vi "Feature Subset Selection (GA).vi"() -> ()   [LabVIEW 2016]
uses:
  _vlib/GA_tParameters.ctl
  4. Accuracy Assessment for EEG Classification/_vlib/CU_ClassifierTypes.ctl
  <vilib>/Math Plots/2D Math Plots/2D Error Bar/2D Error Bar XCtrl/2D Error Bar.xctl
  4. Accuracy Assessment for EEG Classification/_vlib/CU_ClassifierQualityMeasure.ctl
  _vlib/GA_metaParameters.ctl
  <vilib>/vision/Classification.llb/IMAQ SVM Kernel Options.ctl
  <vilib>/Math Plots/2D Math Plots/2D Error Bar/2D Error Bar Datatype/Public/Plot Helper (Fixed).vi
  4. Accuracy Assessment for EEG Classification/Classifier.lvlib
  _vlib/GA.lvlib
  <vilib>/Math Plots/2D Math Plots/2D Error Bar/2D Error Bar Datatype/2D Error Bar Datatype.lvclass
  <vilib>/Analysis/NI_AALBase.lvlib
panel:
  in  "Stop Button":bool
  in  "Tab Control":T1(tab)
  in  "ClassifierQualityMeasure":T2 caption="Критерий оценки точности классификации"
  in  "Use equal number of trials?":bool caption="Включить балансировку классов?"
  in  "Classifier Metaparameter":dbl=5.0 caption="Свободный параметр классификатора" min=0.0 max=100.0 step=0.1 format="%#_2g"
  in  "Iterations Num":i32=5
  in  "Training data paths":path[](array[path]) caption="Пути к файлам с обучающими данными"
  in  "Test data paths":path[](array[path]) caption="Пути к файлам с тестовыми данными"
  in  "True labels for Test data":path[](array[path]) caption="Пути к файлам с метками классов (для тестовых данных)"
  in  "Parameters":T3={"Population size"=100, "Generations no."=20, "Crossover probabality"=0.85, "Mutation mode"=enum."one-point, fixed rate", "Creep mutation"=FALSE, "Mutation rate"=0.05, "Min mutation rate"=0.0005, "Max mutation rate"=0.25, "Relative fitness differential"=1.0, "Reproduction plan"=enum."Steady-state-replace-worst", "Elitism"=FALSE, "FeaturesPerChannel"=5} caption="Параметры генетического алгоритма" {"Relative fitness differential" min=0.0 max=1.0; "Max mutation rate" min=0.0 max=1.0; "Min mutation rate" min=0.0 max=1.0; "Mutation rate" min=0.0 max=1.0; "Crossover probabality" min=0.0 max=1.0; "Generations no." min=1; "Population size" min=1}
  in  "ClassifierType":T4=enum."k NN Classifier" caption="Тип классификатора"
  in  "Start GA":bool
  out "Dataset Num":i32
  out "Total Progress":i32(slide) scale=0.0..25.0
  out "Solution":i32(listbox) caption="Решения, полученные после запусков ГА"
  out "Fitness Chart":cluster{i32[], dbl[]}[](graph) caption="Графики точности классификации"
  out "Accuracies":i32(listbox) caption="Оценки точности классификации на итерациях ГА"
  out "Iteration":i32
  out "Results":string caption="Протокол выполнения программы"
  out "Accuracies out":dbl[][](array[numeric]) caption="Результаты"
  out "2D Error Bar":refnum<class "2D Plot Datatype.lvclass">[](xcontrol) caption="График средней точности классификации"
  # "This VI is a part of BCI Design library, http://www.ru-bci.org \nCopyright © 2020, Sotnikov Peter, All rights reserved. License: GNU GPLv3"
  # "Число запусков ГА для каждого набора данных"
  # "Размер популяции"
  # "Число поколений"
  # "Вероятность скрещивания (кроссовера)"
  # "Тип мутации"
  # "Вероятность мутации"
  # "Значение nu для SVM-классификатора (0,0 .. 1,0)\nЧисло соседей k для kNN-классификатора (1 .. 100)\nЧисло нейронов N скрытого слоя для многослойного персептрона (1 .. 100)"
  # "Минимальная вероятность мутации"
  # "Максимальная вероятность мутации"
  # "Способ включения потомков в популяцию"
  # "Использовать элитизм?"
  # "Общее выполнение"
  # "Набор данных №"
  # "Запуск ГА №"
  # "Среднее \nпо наборам"
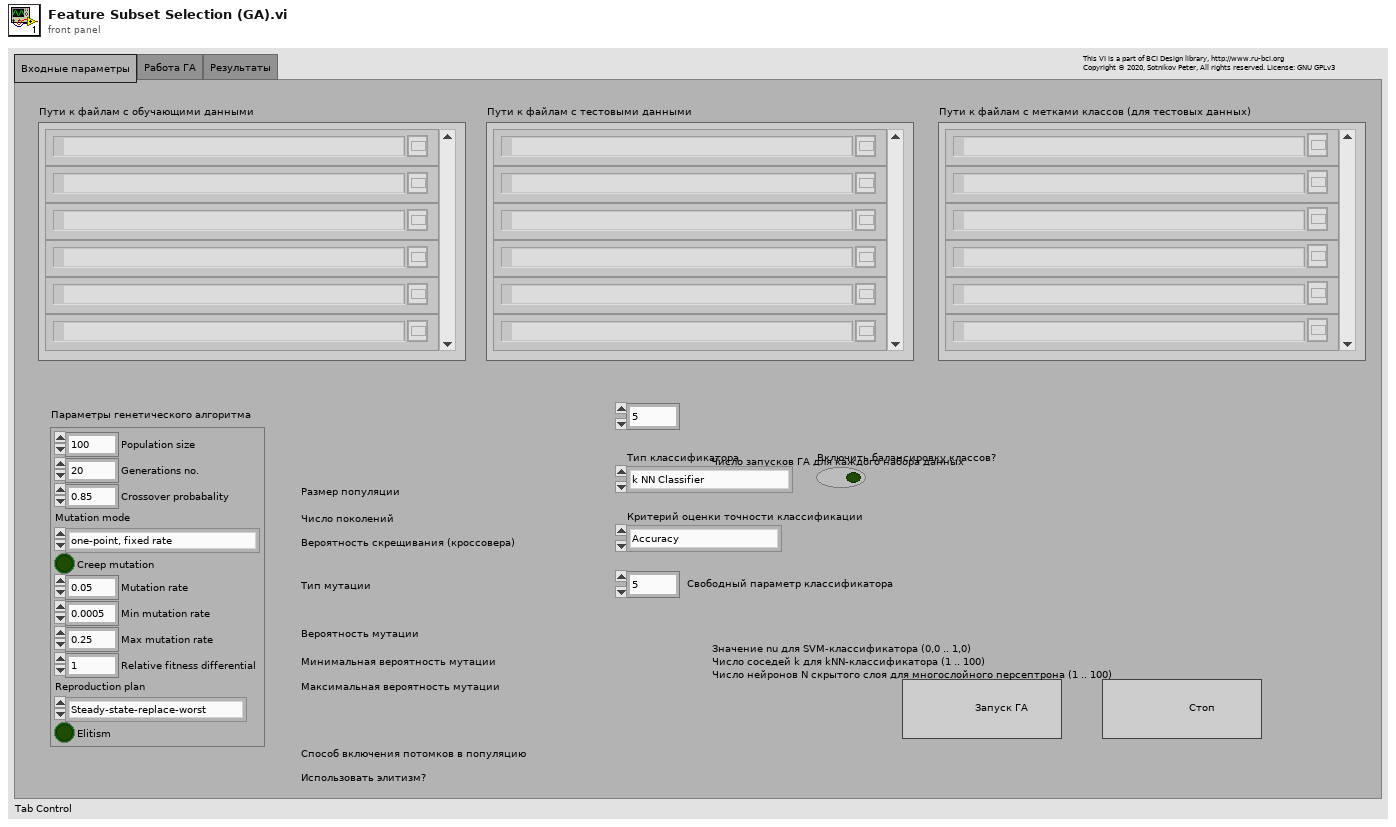
[diagram p1: front panel]
types:
  T1 = enum32{"Входные параметры", "Работа ГА", "Результаты"}
  T2 = typedef "Classifier.lvlib/CU_ClassifierQualityMeasure.ctl" = enum16{"Accuracy", "Cohen's kappa"}
  T3 = typedef "GA.lvlib/GA_tParameters.ctl" = cluster{"Population size":i32, "Generations no.":i32, "Crossover probabality":dbl, "Mutation mode":enum16{"one-point, fixed rate", "one-point, fitness-adjustable rate", "one-point, distance-adjustable rate"}, "Creep mutation":bool, "Mutation rate":dbl, "Min mutation rate":dbl, "Max mutation rate":dbl, "Relative fitness differential":dbl, "Reproduction plan":enum16{"Full generational replacement", "Steady-state-replace-random", "Steady-state-replace-worst"}, "Elitism":bool, "FeaturesPerChannel":i32}
  T4 = typedef "Classifier.lvlib/CU_ClassifierTypes.ctl" = enum16{"Multilayer perceptron", "k NN Classifier", "SVM Committee", "Mahalanobis distance", "SVM Classifier"}
  T5 = typedef "GA.lvlib/GA_metaParameters.ctl" = cluster{"Training Data Path":path, "Test Data Path":path, "True Labels for Test Trials":path, "ClassifierType":T4, "SVM Options":T6, "GA Parameters":T3, "Use equal number of trials?":bool, "Classifier Metaparameter":dbl, "ClassifierQualityMeasure":T2}
  T6 = typedef "IMAQ SVM Kernel Options.ctl" = cluster{"Kernel":enum32{"Linear", "Polynomial", "Gaussian", "RBF"}, "Degree":i32, "Gamma":dbl, "Coefficient":dbl, "Sigma":dbl, "Cache(MB)":dbl}
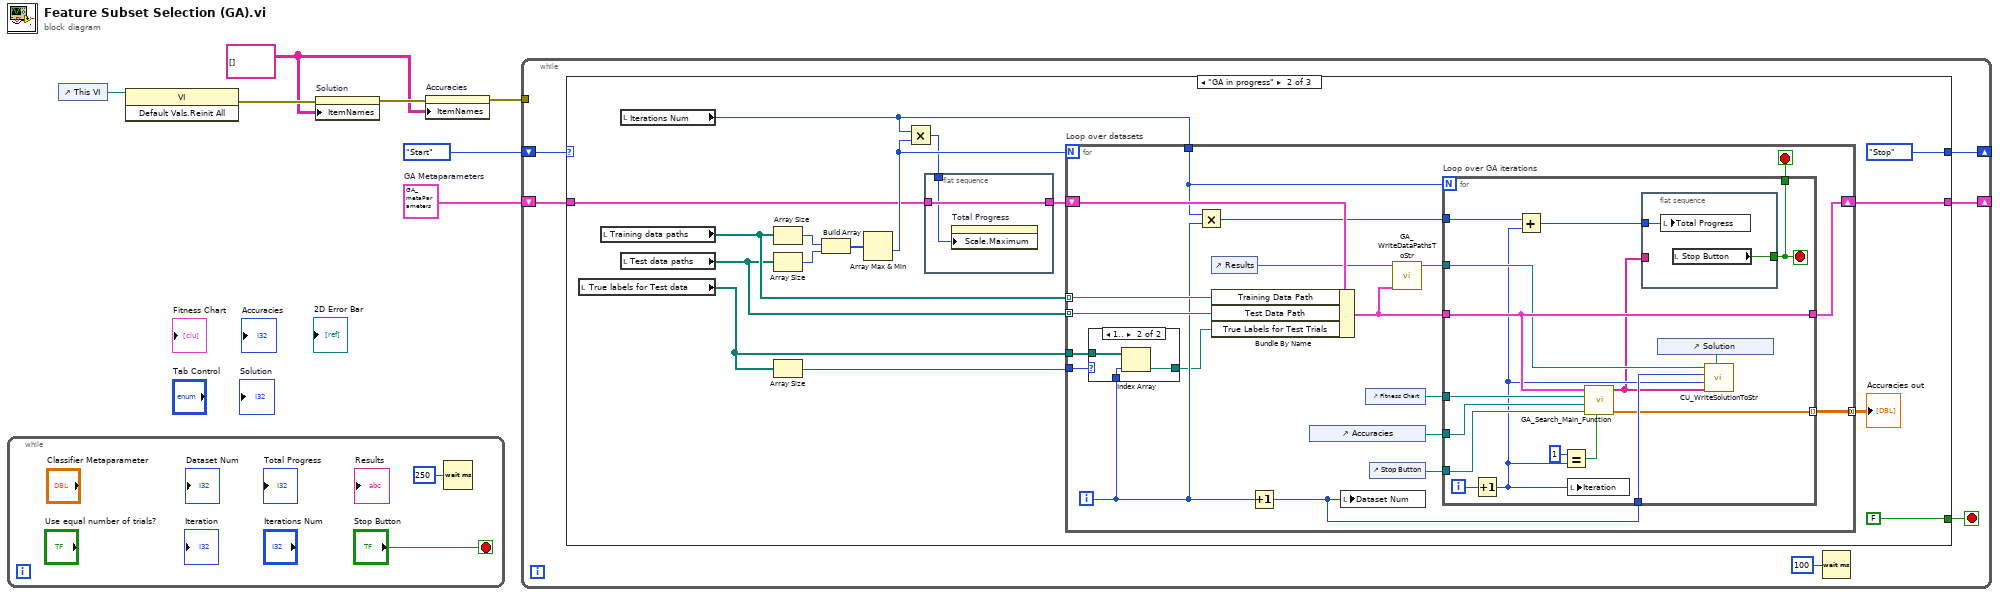
[diagram p0: block diagram]
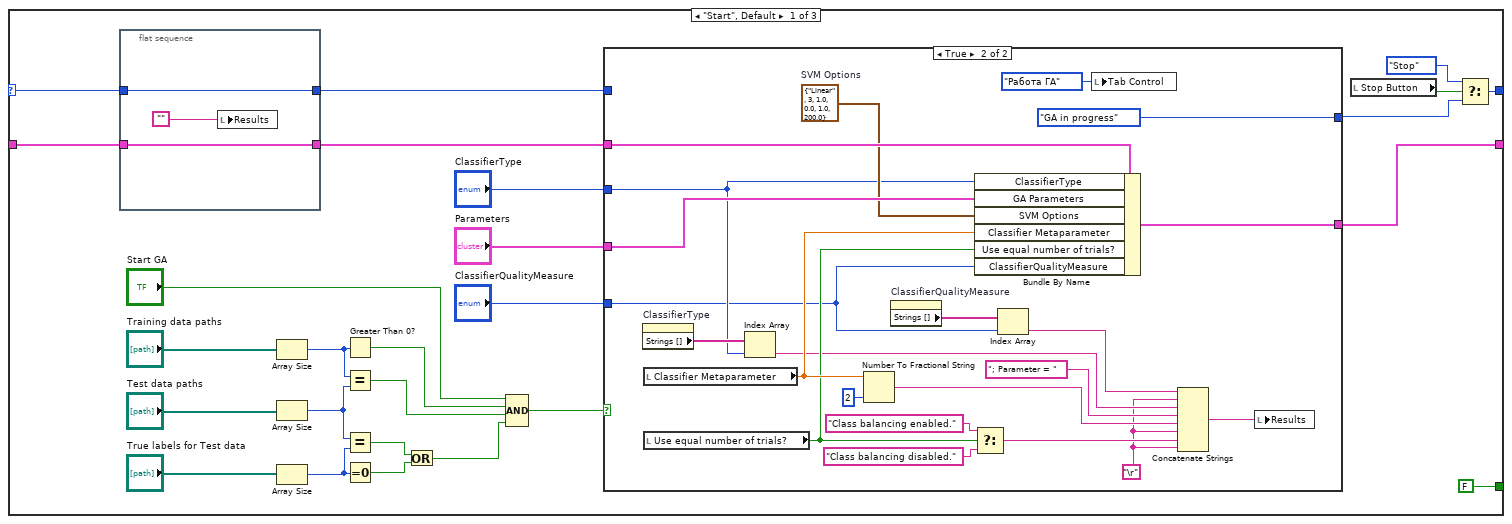
[diagram p2: hidden frame]
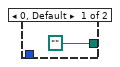
[diagram p4: hidden frame]
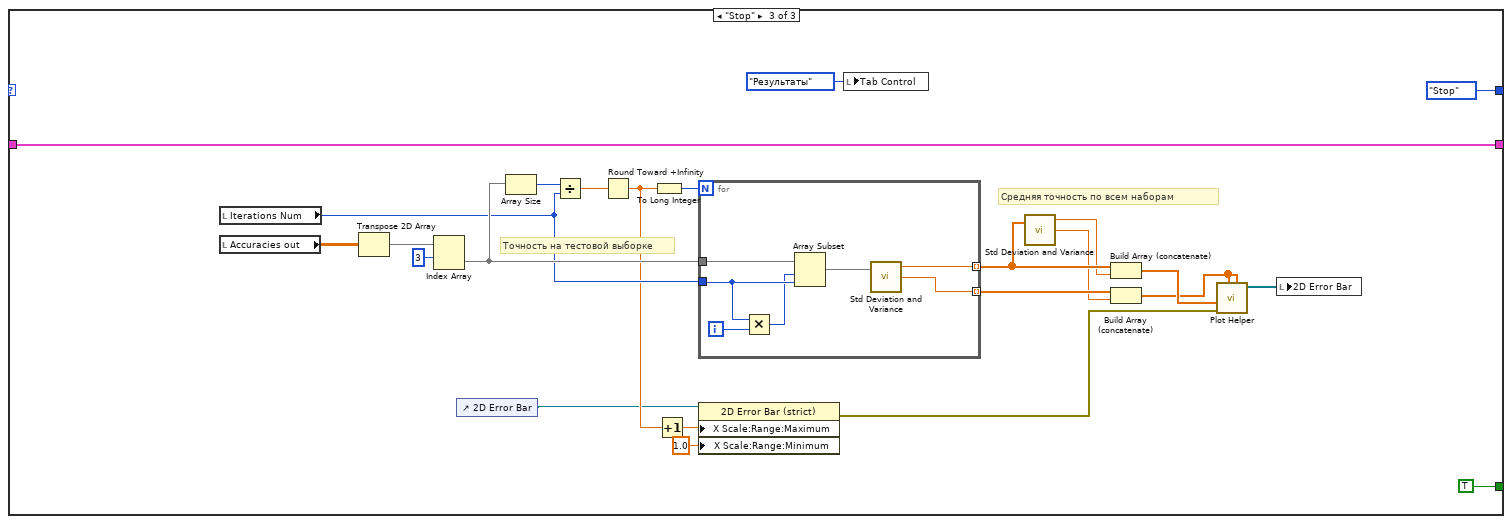
[diagram p5: hidden frame]
diagram:
  w1 = string[][] [] ("Item Names")
  w6 = T5 {"Training Data Path"=path "", "Test Data Path"=path "", "True Labels for Test Trials"=path "", "ClassifierType"=enum."Multilayer perceptron", "SVM Options"={"Kernel"=enum."Linear", "Degree"=0, "Gamma"=0.0, "Coefficient"=0.0, "Sigma"=0.0, "Cache(MB)"=0.0}, "GA Parameters"={"Population size"=0, "Generations no."=0, "Crossover probabality"=0.0, "Mutation mode"=enum."one-point, fixed rate", "Creep mutation"=FALSE, "Mutation rate"=0.0, "Min mutation rate"=0.0, "Max mutation rate"=0.0, "Relative fitness differential"=0.0, "Reproduction plan"=enum."Full generational replacement", "Elitism"=FALSE, "FeaturesPerChannel"=0}, "Use equal number of trials?"=FALSE, "Classifier Metaparameter"=5.0, "ClassifierQualityMeasure"=enum."Accuracy"}  # GA Metaparameters
  n1 = while {
    stop <- "Stop Button" stop-if-true
    n2 = Wait (ms)(milliseconds to wait=u32 250) -> ()  [unwired: 1 out]
  }
  n3 = control-ref of="This VI"() -> (w5:refnum<vi>)
  n4 = invoke class="VI" method="Default Vals.Reinit All"(reference=w5) -> (error out=w4:errorcluster)  [unwired: 2 in, 2 out]
  n5 = property on="Solution" class="MCListbox (strict)"(error in=w4, "ItemNames"=w1) -> (error out=w3:errorcluster)  [unwired: 1 in, 1 out]
  n6 = property on="Accuracies" class="MCListbox (strict)"(error in=w3, "ItemNames"=w1) -> (error out=w2:errorcluster)  [unwired: 1 in, 1 out]
  n7 = while {
    shift-right: [w12] -> _
    shift-left: w6 -> [w14]
    shift-right: [w13] -> _
    shift-left: enum16{"Start", "GA in progress", "Stop"}."Start" -> [w15]
    tunnel: w2 -> [_]
    stop <- w10 stop-if-true
    n8 = case shown="\"GA in progress\"" w15 {
      selector: w15 -> [w27 _ _]
      tunnel: w14 -> [w25 w70 w149]
      tunnel: [w31 enum16{"Start", "GA in progress", "Stop"}."Stop" ("t") enum16{"Start", "GA in progress", "Stop"}."Stop"] -> w13
      tunnel: [w33 w76 w149] -> w12
      tunnel: [FALSE FALSE TRUE] -> w10
      frame "Start", Default {
        n9 = flat-sequence {
          tunnel: w27 -> [w44]
          tunnel: [w44] -> w26
          tunnel: w25 -> [w43]
          tunnel: [w43] -> w24
          frame #0 {
            n10 = local write "Results"("") -> ()
          }
        }
        n11 = Array Size(array="Training data paths") -> (size(s)=w23:i32)
        n12 = Array Size(array="Test data paths") -> (size(s)=w41:i32)
        n13 = Array Size(array="True labels for Test data") -> (size(s)=w22:i32)
        n14 = Greater Than 0?(x=w23) -> (x > 0?=w17:bool)
        n15 = Equal?(x=w23, y=w41) -> (x = y?=w18:bool)
        n16 = Equal?(x=w41, y=w22) -> (x = y?=w21:bool)
        n17 = Equal To 0?(x=w22) -> (x = 0?=w20:bool)
        n18 = Or(x=w21, y=w20) -> (x .or. y?=w19:bool)
        n19 = Compound Arithmetic op=AND("Start GA", w17, w18, w19) -> (w40:bool)
        n20 = case shown="True" w40 {
          tunnel: w24 -> [w46 w68]
          tunnel: "ClassifierType" -> [_ w61]
          tunnel: "Parameters" -> [_ w67]
          tunnel: w26 -> [w45 _]
          tunnel: [w45 enum16{"Start", "GA in progress", "Stop"}."GA in progress"] -> w29
          tunnel: [w46 w64] -> w33
          tunnel: "ClassifierQualityMeasure" -> [_ w48]
          frame False {
          }
          frame True {
            w50 = "\r"
            w66 = T6 {"Kernel"=enum."Linear", "Degree"=3, "Gamma"=1.0, "Coefficient"=0.0, "Sigma"=1.0, "Cache(MB)"=200.0}  # SVM Options
            n21 = property on="ClassifierType" class="Enum (strict)"() -> ("Strings []"=w62:string[])  [unwired: 2 in, 2 out]
            n22 = local read "Classifier Metaparameter"() -> (w59:dbl)
            n23 = local read "Use equal number of trials?"() -> (w57:bool)
            n24 = Index Array(array=w62, index=w61) -> (element=w54:string)
            n25 = Number To Fractional String(number=w59, precision (6)=i16 2) -> (F-format string=w52:string)  [unwired: 2 in]
            n26 = property on="ClassifierQualityMeasure" class="Enum (strict)"() -> ("Strings []"=w49:string[])  [unwired: 2 in, 2 out]
            n27 = Bundle By Name(cluster=w68, "ClassifierType"=w61, "GA Parameters"=w67, "SVM Options"=w66, "Classifier Metaparameter"=w59, "Use equal number of trials?"=w57, "ClassifierQualityMeasure"=w48) -> (w64:T5)
            n28 = Select(t="Class balancing enabled.", s=w57, f="Class balancing disabled.") -> (s? t:f=w51:string)
            n29 = Index Array(array=w49, index=w48) -> (element=w47:string)
            n30 = local write "Tab Control"(T1."Работа ГА" ("Tab Control")) -> ()
            n31 = Concatenate Strings(w47, w50, w54, "; Parameter = ", w52, w50, w51, w50) -> (w60:string)
            n32 = local write "Results"(w60) -> ()
          }
        }
        n33 = local read "Stop Button"() -> (w30:bool)
        n34 = Select(t=enum16{"Start", "GA in progress", "Stop"}."Stop", s=w30, f=w29) -> (s? t:f=w31:enum16{"Start", "GA in progress", "Stop"})
      }
      frame "GA in progress" {
        n35 = local read "True labels for Test data"() -> (w78:path[])
        n36 = local read "Training data paths"() -> (w80:path[])
        n37 = local read "Iterations Num"() -> (w74:i32)
        n38 = local read "Test data paths"() -> (w79:path[])
        n39 = Array Size(array=w80) -> (size(s)=w83:i32)
        n40 = Array Size(array=w79) -> (size(s)=w82:i32)
        n41 = Array Size(array=w78) -> (size(s)=w72:i32)
        n42 = Build Array(w83, w82) -> (w81:i32[])
        n43 = Array Max & Min(array=w81) -> (min value=w73:i32)  [unwired: 3 out]
        n44 = Multiply(x=w74, y=w73) -> (x*y=w69:i32)
        n45 = flat-sequence {
          tunnel: [w86] -> w71
          tunnel: w70 -> [w86]
          tunnel: w69 -> [w85]
          frame #0 {
            n46 = property on="Total Progress" class="Slide (strict)"("Scale.Maximum"=w85) -> ()  [unwired: 2 in, 2 out]
          }
        }
        n47 = for "Loop over datasets" {
          N: w73 -> [_]
          tunnel: w80 -> [w104] mode=indexing
          tunnel: w79 -> [w103] mode=indexing
          tunnel: w78 -> [w88]
          shift-right: [w99] -> w76
          shift-left: w71 -> [w105]
          tunnel: [w97] -> w75 mode=concatenating
          tunnel: w74 -> [w96]
          tunnel: w72 -> [w89]
          i -> [w90]
          stop <- w98 stop-if-true
          n48 = case shown="1.." w89 {
            tunnel: w88 -> [_ w109]
            tunnel: w90 -> [_ w108]
            tunnel: [path "" w107] -> w87
            frame 0, Default {
            }
            frame 1.. {
              n49 = Index Array(array=w109, index=w108) -> (element=w107:path)
            }
          }
          n50 = Multiply(x=w96, y=w90) -> (x*y=w95:i32)
          n51 = control-ref of="Results"() -> (w94:refnum<vi>)
          n52 = Bundle By Name(cluster=w105, "Training Data Path"=w104, "Test Data Path"=w103, "True Labels for Test Trials"=w87) -> (w92:T5)
          n53 = Increment(x=w90) -> (x+1=w91:i32)
          n54 = control-ref of="Accuracies"() -> (w101:refnum<vi>)
          n55 = local write "Dataset Num"(w91) -> ()
          n56 = control-ref of="Fitness Chart"() -> (w102:refnum<vi>)
          n57 = control-ref of="Stop Button"() -> (w100:refnum<vi>)
          n58 = call "GA_WriteDataPathsToStr.vi"("GA Metaparameters in"=w92, "String Ref in"=w94) -> ("String Ref out"=w93:refnum<vi>)  [unwired: 7 in, 2 out]
          n59 = for "Loop over GA iterations" {
            N: w96 -> [_]
            tunnel: w92 -> [w122]
            tunnel: w102 -> [w125]
            tunnel: w101 -> [w124]
            tunnel: w100 -> [w123]
            tunnel: [w111] -> w97 mode=indexing
            tunnel: [w122] -> w99
            tunnel: [w121] -> w98
            tunnel: w95 -> [w120]
            tunnel: w93 -> [w117]
            tunnel: w91 -> [w115]
            i -> [w119]
            stop <- w121 stop-if-true
            n60 = Increment(x=w119) -> (x+1=w114:i32)
            n61 = Add(x=w120, y=w114) -> (x+y=w118:i32)
            n62 = Equal?(x=1, y=w114) -> (x = y?=w112:bool)
            n63 = local write "Iteration"(w114) -> ()
            n64 = call "GA_Search_Main_Function.vi"("ReInitialize?"=w112, "Stop ButtonRef in"=w123, "Accuracies Listbox Ref in"=w124, "Fitness Chart Ref in"=w125, "GA Metaparameters in"=w122) -> ("Accuracies out (double)"=w111:dbl[], "Accuracies out (string)"=w110:string[])  [unwired: 5 in]
            n65 = flat-sequence {
              tunnel: [w127] -> w121
              tunnel: w118 -> [w126]
              tunnel: w110 -> [_]
              frame #0 {
                n66 = local write "Total Progress"(w126) -> ()
                n67 = local read "Stop Button"() -> (w127:bool)
              }
            }
            n68 = control-ref of="Solution"() -> (w116:refnum<vi>)
            n69 = call "CU_WriteSolutionToStr.vi"("ListBox Ref in"=w116, "Solution in"=w110, "Iteration Num"=w114, "Dataset Num"=w115, "String Ref in"=w117) -> ()  [unwired: 5 in, 2 out]
          }
        }
        "Accuracies out" <- w75
      }
      frame "Stop" {
        # "Средняя точность по всем наборам"
        # "Точность на тестовой выборке"
        n70 = local read "Iterations Num"() -> (w142:i32)
        n71 = local read "Accuracies out"() -> (w148:dbl[][])
        n72 = Transpose 2D Array(2D array=w148) -> (transposed array=w147:dbl[][])
        n73 = Index Array(array=w147, index (row)=3) -> (element=w143:dbl[])  [unwired: 1 in]
        n74 = control-ref of="2D Error Bar"() -> (w129:refnum<vi>)
        n75 = Array Size(array=w143) -> (size(s)=w145:i32)
        n76 = Divide(x=w145, y=w142) -> (x/y=w144:dbl)
        n77 = Round Toward +Infinity(x=w144) -> (ceil(x): smallest int >= x=w131:dbl)
        n78 = To Long Integer(number=w131) -> (32bit integer=w132:i32)
        n79 = Increment(x=w131) -> (x+1=w134:dbl)
        n80 = for {
          N: w132 -> [_]
          tunnel: w143 -> [w158]
          tunnel: w142 -> [w157]
          tunnel: [w154] -> w141 mode=indexing
          tunnel: [w153] -> w139 mode=indexing
          i -> [w152]
          n81 = Multiply(x=w157, y=w152) -> (x*y=w156:i32)
          n82 = Array Subset(array=w158, index=w156, length=w157) -> (w155:dbl[])
          n83 = call <vilib>:"Std Deviation and Variance.vi"("X"=w155) -> ("mean"=w154:dbl, "standard deviation"=w153:dbl)  [unwired: 1 in, 1 out]
        }
        n84 = property class="2D Error Bar (strict)"(reference=w129, "X Scale:Range:Maximum"=w134, "X Scale:Range:Minimum"=1.0) -> (error out=w133:errorcluster)  [unwired: 1 in, 1 out]
        n85 = local write "Tab Control"(T1."Результаты" ("Tab Control")) -> ()
        n86 = call <vilib>:"Std Deviation and Variance.vi"("X"=w141) -> ("mean"=w140:dbl, "standard deviation"=w138:dbl)  [unwired: 1 in, 1 out]
        n87 = Build Array (concatenate)(w141, w140) -> (w137:dbl[])
        n88 = Build Array (concatenate)(w139, w138) -> (w136:dbl[])
        n89 = call-poly <vilib>:"Plot Helper.vi"("error b vector"=w136, "error a vector"=w136, "error in (no error)"=w133, "y vector"=w137) -> ("2D Plot Class Obj Array out"=w135:refnum<class "2D Plot Datatype.lvclass">[])  [unwired: 2 in, 5 out]
        n90 = local write "2D Error Bar"(w135) -> ()
      }
    }
    n91 = Wait (ms)(milliseconds to wait=u32 100) -> ()  [unwired: 1 out]
  }
